vi "ff wframe.vi"(10 "frame_raw":u8[][](array[numeric])) -> (2 "function return":i32)   [LabVIEW 2013, in "ffvi.lvlib"]
doc: "int ff_wframe(void *frame_raw);"
uses:
  ffvi.lvlib
  ffvi.dll
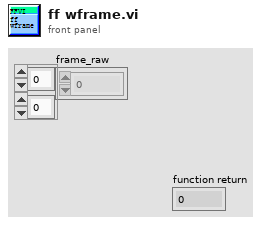
[diagram p1: front panel]
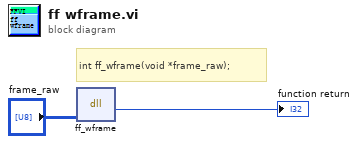
[diagram p0: block diagram]
diagram:
  # "int ff_wframe(void *frame_raw);"
  n1 = dll-call lib="D:/ffmpeg/ffvi/ffvi.*" fn="ff_wframe"("frame_raw"="frame_raw") -> ("return type"=→"function return":i32)  [unwired: 4 in, 2 out]
